vi "MES.main.xio.vi"() -> ()   [LabVIEW 2018]
uses:
  Ctl.xio/type defs/ini file actions.ctl
  Ctl.xio/type defs/ini entry value.ctl
  Ctl.xio/type defs/ini entry.ctl
  Ctl.xio/type defs/ini entry types.ctl
  <vilib>/Utility/file.llb/Read From Spreadsheet File (string).vi
panel:
  out "Ver":string
  in  "退出系统":bool
  in  "自定义标签":bool
  out "项目名称":string
  in  "用户登录":bool
  in  "Buttons":T1
  in  "分站":T2(tab)
  out "粗切工位生产信息":string[][](table)
  out "热处理工位生产信息":string[][](table)
  out "精切工位生产信息":string[][](table)
  out "PDF焊接工位生产信息":string[][](table)
  out "打凹点\\预载力工位生产信息":string[][](table)
  out "收卷工位生产信息":string[][](table)=[["CCFA1I001", "", "", "", "", "", "", "", "", "", "", "", "", "", "", "", "", "", "", "", "", "", "", "", "", "", "", "", "", "", "", "", ""], ["CCFA1Y000", "V254ACCFA1BB092308232129", "2023.08.23 21:29:24", "CCFA1BB09", "V254A   .OUT", "50", "35", "500", "20", "2", "V254A", "V254ACCFA1BB092308232129", "2023.08.23 21:35:37", "CCFA1BB09", "V254A   .OUT", "23", "13", "500", "5", "2", "V254A", "CCFA1Y000", "V254ACCFA1BB092308232129", "", "", "", "", "", "", "", "", "", ""]]
  out "EOL检测工位生产信息":string[][](table)
  out "status 5":bool
  out "status 6":bool
  out "status 3":bool
  out "status 4":bool
  out "收卷当期项目":string
  out "PDF项目":string
  out "精切项目":string
  out "热处理项目":string
  out "EOL 终检条码（未启用）":string
  out "EOL 当前状态":string
  out "收卷当前状态":string
  out "收卷上料车条码":string
  out "PDF焊接固化料车条码":string
  out "PDF当前状态":string
  out "PDF焊接上料车条码":string
  out "精切当前状态":string
  out "精切下料车条码":string
  out "精切上料车条码":string
  in  "当前项目选择":u16(ring) items=["V254A", "V254B", "C101A", "C101B", "FS11A", "FS11B", "FS11C", "V254C", "V254D", "F78", "V254T1", "F78", "F78B", "V2541700"]
  out "热处理当前状态":string
  out "热处理出口条码":string
  out "热处理入口条码":string
  out "粗切当前状态":string
  out "粗切条码":string
  out "粗切项目":string
  out "status 1":bool
  out "status 2":bool
  out "当前时间":string
  out "当前日期":string
  # "汽车遮阳帘生产线"
  # "当前项目"
  # "当前项目"
  # "当前项目"
  # "当前项目"
  # "当前项目"
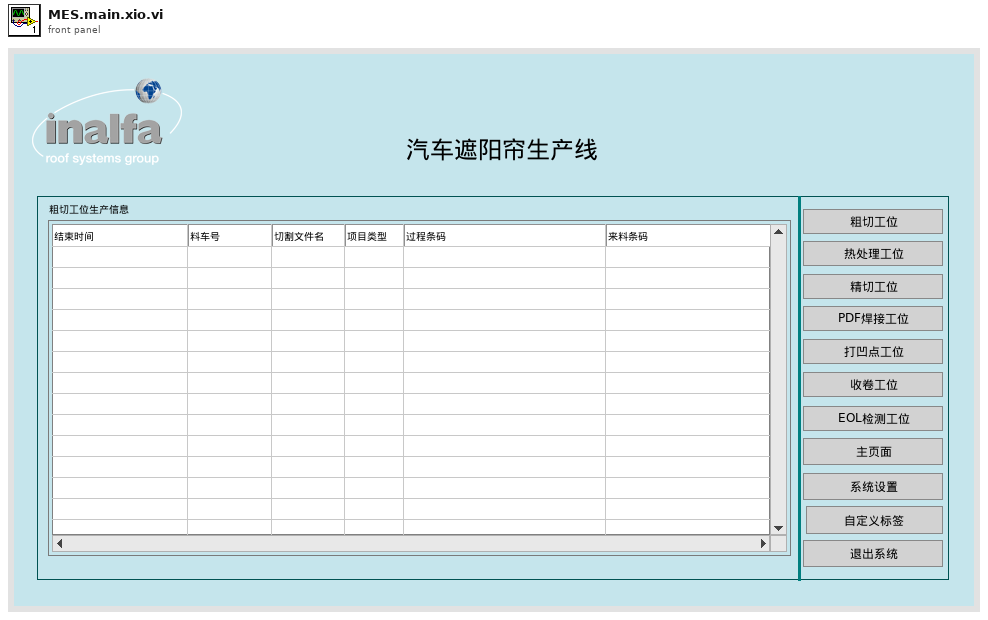
[diagram p1: front panel]
types:
  T1 = cluster{"粗切工位":bool, "热处理工位":bool, "精切工位":bool, "PDF焊接工位":bool, "打凹点工位":bool, "收卷工位":bool, "EOL检测工位":bool, "工位预览":bool}
  T2 = enum32{"粗切工位", "热处理工位", "精切工位", "PDF焊接工位", "打凹点\\预载力工位", "收卷工位", "EOL检测工位", "所有工位预览"}
  T3 = enum32{"产品配置", "粗切工位", "热处理工位", "精切工位", "PDF焊接工位", "打凹点\\预载力工位", "收卷工位", "EOL检测工位", "所有工位预览"}
  T4 = typedef "ini entry.ctl" = cluster{"section":string, "key":string, "type":T5, "default value":T6}
  T5 = typedef "ini entry types.ctl" = enum16{"Boolean", "Double", "I32", "Path", "String", "U32"}
  T6 = typedef "ini entry value.ctl" = cluster{"Boolean":bool, "Dbl":dbl, "I32":i32, "Path":path, "String":string, "U32":u32}
  T7 = typedef "ini file actions.ctl" = enum16{"read ini", "write ini"}
  T8 = cluster{"打凹点\\预载力工位生产信息":refnum<vi>, "项目名称":refnum<vi>}
  T9 = cluster{"粗切工位生产信息":refnum<vi>, "粗切条码":refnum<vi>, "粗切当前状态":refnum<vi>, "粗切项目":refnum<vi>, "status 1":refnum<vi>}
  T10 = cluster{"热处理工位生产信息":refnum<vi>, "热处理入口条码":refnum<vi>, "热处理当前状态":refnum<vi>, "热处理出口条码":refnum<vi>, "热处理项目":refnum<vi>, "status 2":refnum<vi>}
  T11 = cluster{"精切工位生产信息":refnum<vi>, "精切上料车条码":refnum<vi>, "精切当前状态":refnum<vi>, "精切下料车条码":refnum<vi>, "精切项目":refnum<vi>, "status 3":refnum<vi>}
  T12 = cluster{"PDF焊接工位生产信息":refnum<vi>, "PDF焊接上料车条码":refnum<vi>, "PDF当前状态":refnum<vi>, "PDF焊接固化料车条码":refnum<vi>, "PDF项目":refnum<vi>, "status 4":refnum<vi>}
  T13 = cluster{"EOL检测工位生产信息":refnum<vi>, "EOL 终检条码（未启用）":refnum<vi>, "EOL 当前状态":refnum<vi>, "项目名称":refnum<vi>, "status 6":refnum<vi>}
  T14 = cluster{"收卷工位生产信息":refnum<vi>, "收卷上料车条码":refnum<vi>, "收卷当前状态":refnum<vi>, "收卷当期项目":refnum<vi>, "status 5":refnum<vi>}
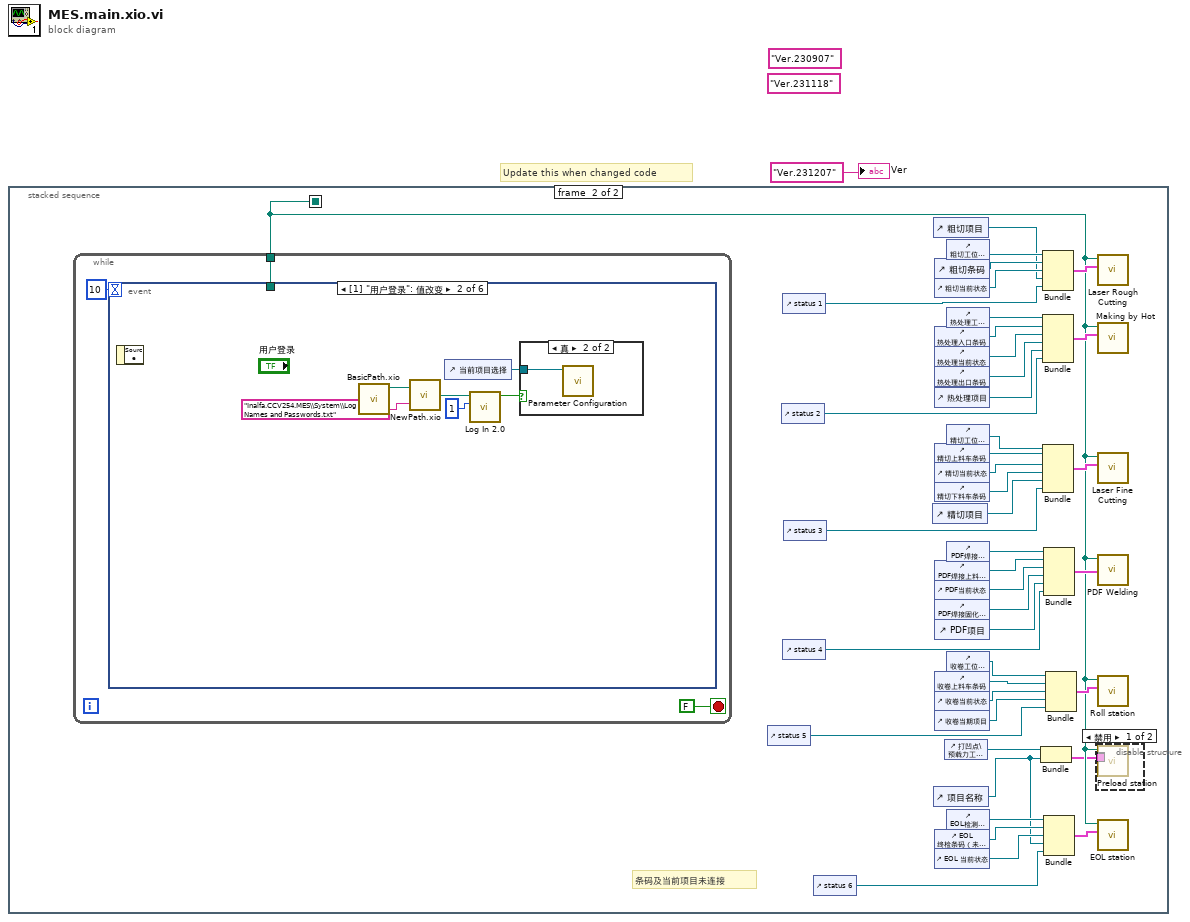
[diagram p0: block diagram]
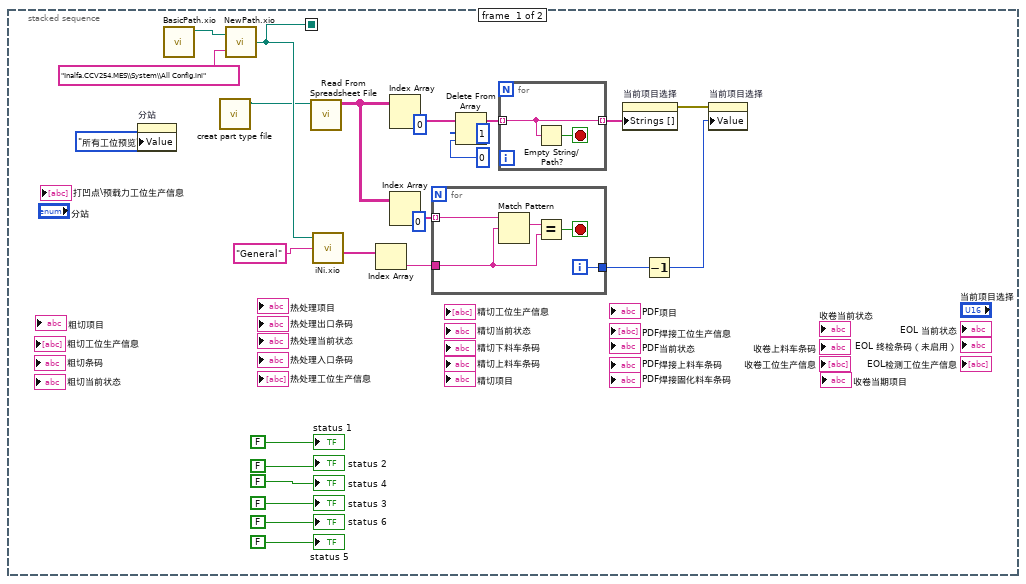
[diagram p2: hidden frame]
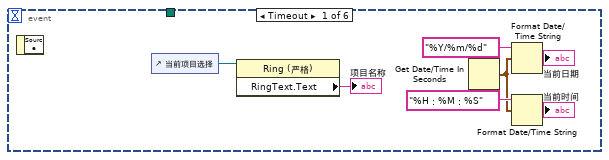
[diagram p4: hidden frame]
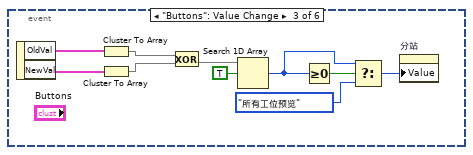
[diagram p6: hidden frame]
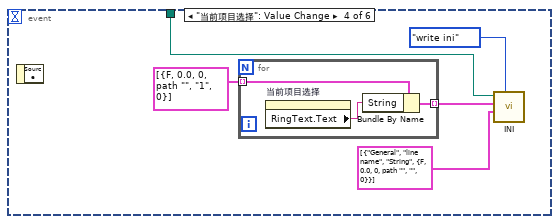
[diagram p7: hidden frame]
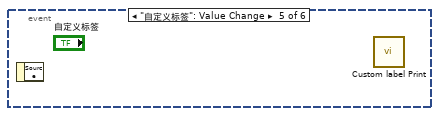
[diagram p8: hidden frame]
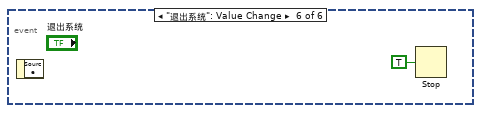
[diagram p9: hidden frame]
diagram:
  (unwired) "Ver.231118" ("Ver")
  (unwired) "Ver.230907" ("Ver")
  # "Update this when changed code"
  n1 = stacked-sequence {
    seq-local: [w19 _] -> [_ w43]
    frame #0 {
      n2 = property on="分站" class="TabCtl (严格)"("Value"=T2."所有工位预览" ("分站")) -> ()  [unwired: 2 in, 2 out]
      n3 = call "BasicPath.xio.vi"() -> ("stripped path"=w26:path)  [unwired: 10 in, 1 out]
      n4 = call "creat part type file.vi"() -> ("new file path (Not A Path if cancelled)"=w8:path)  [unwired: 11 in]
      n5 = call "NewPath.xio.vi"("Append path"="Inalfa.CCV254.MES\\System\\All Config.ini", "Basic path"=w26) -> ("New path"=w19:path)
      n6 = call-poly <vilib>:"Read From Spreadsheet File.vi"("file path (dialog if empty)"=w8) -> ("all rows"=w12:string[][])  [unwired: 6 in, 4 out]
      n7 = call "iNi.xio.vi"("configuration file path"=w19, "Sections"="General") -> ("Values"=w21:string[])  [unwired: 1 in, 4 out]
      n8 = Index Array(array=w21) -> (element=w23:string)  [unwired: 1 in]
      n9 = Index Array(array=w12, index (col)=0 ("禁用的索引 (列)")) -> (element=w15:string[])  [unwired: 1 in]
      n10 = Index Array(array=w12, index (col)=0 ("禁用的索引 (列)")) -> (element=w24:string[])  [unwired: 1 in]
      n11 = for {
        tunnel: w24 -> [w34] mode=indexing
        tunnel: [w31] -> w25
        tunnel: w23 -> [w30]
        i -> [w31]
        stop <- w32 stop-if-true
        n12 = Match Pattern(string=w34, regular expression=w30) -> (match substring=w33:string)  [unwired: 1 in, 3 out]
        n13 = Equal?(x=w33, y=w30) -> (x = y?=w32:bool)
      }
      n14 = Delete From Array(array=w15, length=1 ("长度"), index=0 ("索引")) -> (array with subset deleted=w13:string[])  [unwired: 1 out]
      n15 = for {
        tunnel: w13 -> [w28] mode=indexing
        tunnel: [w28] -> w9 mode=indexing
        stop <- w29 stop-if-true
        n16 = Empty String/Path?(string/path=w28) -> (empty?=w29:bool)
      }
      n17 = property on="当前项目选择" class="Ring (严格)"("Strings []"=w9) -> (error out=w11:errorcluster)  [unwired: 2 in, 1 out]
      n18 = Decrement(x=w25) -> (x-1=w10:i32)
      n19 = property on="当前项目选择" class="Ring (严格)"(error in=w11, "Value"=w10) -> ()  [unwired: 1 in, 2 out]
      "status 2" <- FALSE ("status 2")
      "status 4" <- FALSE ("status 4")
      "status 3" <- FALSE ("status 3")
      "status 6" <- FALSE ("status 6")
      "status 5" <- FALSE ("status 5")
      "status 1" <- FALSE ("status 1")
    }
    frame #1 {
      # "条码及当前项目未连接"
      n20 = while {
        tunnel: w43 -> [w79]
        stop <- FALSE stop-if-true
        n21 = event shown="[1] \"用户登录\": 值改变" {
          selector: _ -> [_ _ _ _ _ _]
          dyn-events: _ -> [_ _ _ _ _ _]
          timeout: 10 -> [_ _ _ _ _ _]
          tunnel: w79 -> [_ _ _ w106 _ _]
          event Timeout {
            n22 = event-data() -> ()  [unwired: 1 in, 1 out]
            n23 = control-ref of="当前项目选择"() -> (w83:refnum<vi>)
            n24 = property class="Ring (严格)"(reference=w83) -> ("RingText.Text"=→"项目名称":string)  [unwired: 1 in, 2 out]
            n25 = Get Date/Time In Seconds() -> (seconds since 1Jan1904=w87:timestamp)
            n26 = Format Date/Time String(time format string (%c)="%Y/%m/%d" ("时间格式字符串(%c)"), seconds (now)=w87) -> (date/time string=→"当前日期":string)  [unwired: 1 in]
            n27 = Format Date/Time String(time format string (%c)="%H：%M：%S" ("时间格式字符串(%c)"), seconds (now)=w87) -> (date/time string=→"当前时间":string)  [unwired: 1 in]
          }
          event "用户登录": Value Change {
            n28 = event-data() -> ()  [unwired: 1 in, 1 out]
            n29 = call "BasicPath.xio.vi"() -> ("stripped path"=w93:path)  [unwired: 10 in, 1 out]
            n30 = call "NewPath.xio.vi"("Append path"="Inalfa.CCV254.MES\\System\\Log In\\User Names and Passwords.txt", "Basic path"=w93) -> ("New path"=w92:path)
            n31 = control-ref of="当前项目选择"() -> (w89:refnum<vi>)
            n32 = call "Log In 2.0.vi"("required access level"=1, "Program Root Path"=w92) -> ("passed"=w90:bool)  [unwired: 6 in, 3 out]
            n33 = case shown="真" w90 {
              tunnel: w89 -> [_ w95]
              frame False {
              }
              frame True {
                n34 = call "Parameter Configuration.vi"("当前项目选择"=w95) -> ()  [unwired: 11 in]
              }
            }
          }
          event "Buttons": Value Change {
            n35 = event-data() -> ("OldVal"=w105:T1, "NewVal"=w104:T1)  [unwired: 1 in]
            n36 = Cluster To Array(cluster=w105) -> (array=w103:bool[])
            n37 = Cluster To Array(cluster=w104) -> (array=w102:bool[])
            n38 = Exclusive Or(1:w102, 2:w103) -> (0:w101:bool[])
            n39 = Search 1D Array(1D array=w101, element=TRUE) -> (index of element=w96:i32)  [unwired: 1 in]
            n40 = Greater Or Equal To 0?(x=w96) -> (x >= 0?=w99:bool)
            n41 = Select(t=w96, s=w99, f=T3."所有工位预览" ("分站")) -> (s? t:f=w98:u32)
            n42 = property on="分站" class="TabCtl (严格)"("Value"=w98) -> ()  [unwired: 2 in, 2 out]
          }
          event "当前项目选择": Value Change {
            n43 = event-data() -> ()  [unwired: 1 in, 1 out]
            n44 = for {
              tunnel: T6[] [{"Boolean"=FALSE, "Dbl"=0.0, "I32"=0, "Path"=path "", "String"="1", "U32"=0}] ("values in") -> [w113] mode=indexing
              tunnel: [w111] -> w107 mode=indexing
              n45 = property on="当前项目选择" class="Ring (严格)"() -> ("RingText.Text"=w112:string)  [unwired: 2 in, 2 out]
              n46 = Bundle By Name(cluster=w113, "String"=w112) -> (w111:T6)
            }
            n47 = call "INI.vi"("configuration file path"=w106, "action"=ini_file_actions."write ini", "values in"=w107, "ini entry descriptors"=T4[] [{"section"="General", "key"="line name", "type"=enum."String", "default value"={"Boolean"=FALSE, "Dbl"=0.0, "I32"=0, "Path"=path "", "String"="", "U32"=0}}]) -> ()  [unwired: 2 in, 3 out]
          }
          event "自定义标签": Value Change {
            n48 = event-data() -> ()  [unwired: 1 in, 1 out]
            n49 = call "Custom label Print.vi"() -> ()  [unwired: 12 in]
          }
          event "退出系统": Value Change {
            n50 = event-data() -> ()  [unwired: 1 in, 1 out]
            n51 = Stop(stop? (T)=TRUE ("停止？(T)")) -> ()
          }
        }
      }
      n52 = control-ref of="status 5"() -> (w35:refnum<vi>)
      n53 = control-ref of="status 2"() -> (w39:refnum<vi>)
      n54 = control-ref of="status 1"() -> (w40:refnum<vi>)
      n55 = control-ref of="status 4"() -> (w37:refnum<vi>)
      n56 = control-ref of="status 3"() -> (w38:refnum<vi>)
      n57 = control-ref of="status 6"() -> (w36:refnum<vi>)
      n58 = control-ref of="精切项目"() -> (w49:refnum<vi>)
      n59 = control-ref of="粗切项目"() -> (w45:refnum<vi>)
      n60 = control-ref of="项目名称"() -> (w41:refnum<vi>)
      n61 = control-ref of="粗切条码"() -> (w75:refnum<vi>)
      n62 = control-ref of="粗切当前状态"() -> (w74:refnum<vi>)
      n63 = control-ref of="热处理入口条码"() -> (w73:refnum<vi>)
      n64 = control-ref of="热处理当前状态"() -> (w71:refnum<vi>)
      n65 = control-ref of="热处理出口条码"() -> (w70:refnum<vi>)
      n66 = control-ref of="热处理项目"() -> (w48:refnum<vi>)
      n67 = control-ref of="精切上料车条码"() -> (w67:refnum<vi>)
      n68 = control-ref of="精切当前状态"() -> (w66:refnum<vi>)
      n69 = control-ref of="精切下料车条码"() -> (w65:refnum<vi>)
      n70 = control-ref of="PDF焊接上料车条码"() -> (w61:refnum<vi>)
      n71 = control-ref of="PDF当前状态"() -> (w60:refnum<vi>)
      n72 = control-ref of="PDF焊接固化料车条码"() -> (w58:refnum<vi>)
      n73 = control-ref of="PDF项目"() -> (w47:refnum<vi>)
      n74 = control-ref of="收卷上料车条码"() -> (w55:refnum<vi>)
      n75 = control-ref of="收卷当前状态"() -> (w54:refnum<vi>)
      n76 = control-ref of="收卷当期项目"() -> (w46:refnum<vi>)
      n77 = control-ref of="EOL 终检条码（未启用）"() -> (w50:refnum<vi>)
      n78 = control-ref of="EOL 当前状态"() -> (w51:refnum<vi>)
      n79 = control-ref of="打凹点\\预载力工位生产信息"() -> (w44:refnum<vi>)
      n80 = control-ref of="粗切工位生产信息"() -> (w76:refnum<vi>)
      n81 = control-ref of="热处理工位生产信息"() -> (w72:refnum<vi>)
      n82 = control-ref of="精切工位生产信息"() -> (w63:refnum<vi>)
      n83 = control-ref of="PDF焊接工位生产信息"() -> (w62:refnum<vi>)
      n84 = control-ref of="收卷工位生产信息"() -> (w56:refnum<vi>)
      n85 = control-ref of="EOL检测工位生产信息"() -> (w52:refnum<vi>)
      n86 = Bundle("打凹点\\预载力工位生产信息"=w44, "项目名称"=w41) -> (w42:T8)  [unwired: 1 in]
      n87 = Bundle("粗切工位生产信息"=w76, "粗切条码"=w75, "粗切当前状态"=w74, "粗切项目"=w45, "status 1"=w40) -> (w69:T9)  [unwired: 1 in]
      n88 = Bundle("热处理工位生产信息"=w72, "热处理入口条码"=w73, "热处理当前状态"=w71, "热处理出口条码"=w70, "热处理项目"=w48, "status 2"=w39) -> (w68:T10)  [unwired: 1 in]
      n89 = Bundle("精切工位生产信息"=w63, "精切上料车条码"=w67, "精切当前状态"=w66, "精切下料车条码"=w65, "精切项目"=w49, "status 3"=w38) -> (w64:T11)  [unwired: 1 in]
      n90 = Bundle("PDF焊接工位生产信息"=w62, "PDF焊接上料车条码"=w61, "PDF当前状态"=w60, "PDF焊接固化料车条码"=w58, "PDF项目"=w47, "status 4"=w37) -> (w59:T12)  [unwired: 1 in]
      n91 = Bundle("EOL检测工位生产信息"=w52, "EOL 终检条码（未启用）"=w50, "EOL 当前状态"=w51, "项目名称"=w41, "status 6"=w36) -> (w53:T13)  [unwired: 1 in]
      n92 = Bundle("收卷工位生产信息"=w56, "收卷上料车条码"=w55, "收卷当前状态"=w54, "收卷当期项目"=w46, "status 5"=w35) -> (w57:T14)  [unwired: 1 in]
      n93 = disable-structure shown="禁用" {
        disable-tunnel: w43 -> [w78 _]
        disable-tunnel: w42 -> [w77 _]
        frame Disabled {
          n94 = call "Preload station.vi"("configuration file path"=w78, "Preload station msic inf"=w77) -> ()  [unwired: 4 in]
        }
        frame Enabled {
        }
      }
      n95 = call "Laser Rough Cutting.vi"("configuration file path"=w43, "rough cutting msic"=w69) -> ()  [unwired: 4 in]
      n96 = call "Making by Hot.vi"("configuration file path"=w43, "making by hot msic inf"=w68) -> ()  [unwired: 4 in]
      n97 = call "Laser Fine Cutting.vi"("configuration file path"=w43, "fine cutting msic"=w64) -> ()  [unwired: 4 in]
      n98 = call "PDF Welding.vi"("configuration file path"=w43, "PDF Welding msic inf"=w59) -> ()  [unwired: 4 in]
      n99 = call "Roll station.vi"("configuration file path"=w43, "Roll station msic inf"=w57) -> ()  [unwired: 4 in]
      n100 = call "EOL station.vi"("configuration file path"=w43, "EOL station msic inf"=w53) -> ()  [unwired: 4 in]
    }
  }
  "Ver" <- "Ver.231207" ("Ver")
